vi "hextstr.vi"(2 "new element/subarray":i32, 3 "index":i32=4, 4 "Array":i32[](array[numeric])=[32, 40, 63, 0, 0, 9, 156, 255, 10, 0]) -> (0 "hex integer string":string[](array[string]), 1 "String":string)   [LabVIEW 2017]
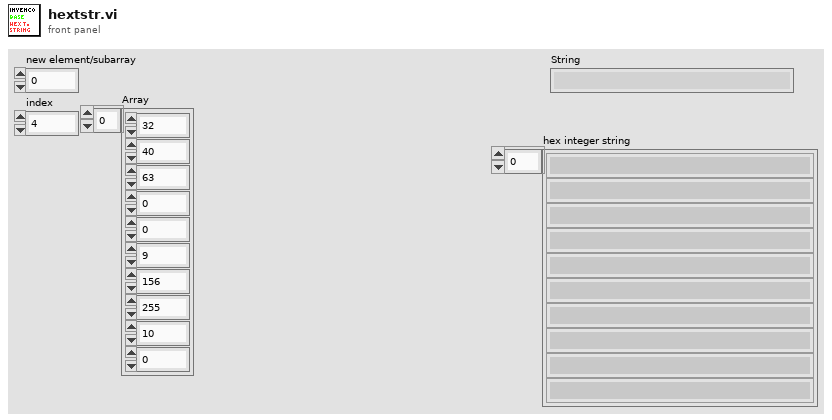
[diagram p1: front panel]
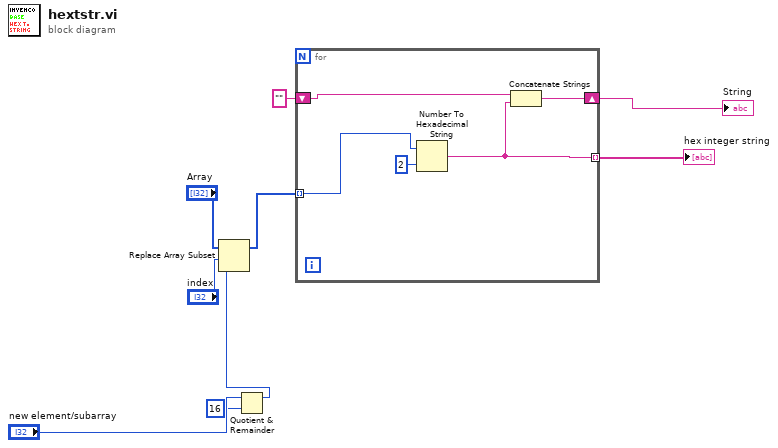
[diagram p0: block diagram]
diagram:
  n1 = Quotient & Remainder(x="new element/subarray", y=16) -> (x-y*floor(x/y)=w2:i32)  [unwired: 1 out]
  n2 = Replace Array Subset(array="Array", new element=w2, index="index") -> (w8:i32[])
  n3 = for {
    tunnel: [w12] -> w9 mode=indexing
    tunnel: w8 -> [w13] mode=indexing
    shift-right: [w11] -> w1
    shift-left: "" -> [w10]
    n4 = Number To Hexadecimal String(1:i16 2 ("width (-)"), 2:w13) -> (0:w12:string)
    n5 = Concatenate Strings(w10, w12) -> (w11:string)
  }
  "hex integer string" <- w9
  "String" <- w1
